vi "Read X.vi"(8 "error in (no error)":errorcluster, 11 "Vec3d Class in":refnum<class "Vec3d Class.lvclass">) -> (0 "error out":errorcluster, 2 "X":dbl, 3 "Vec3d Class out":refnum<class "Vec3d Class.lvclass">)   [LabVIEW 2011, in "Vec3d Class.lvclass"]
uses:
  Vec3d Class.lvclass
  Vec3d Class.lvclass/Vec3d Class.ctl
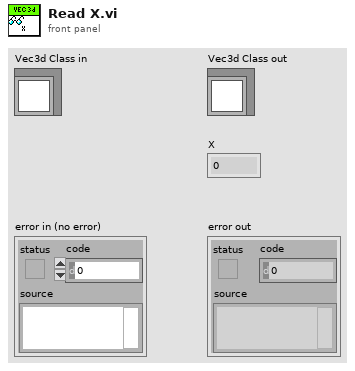
[diagram p1: front panel]
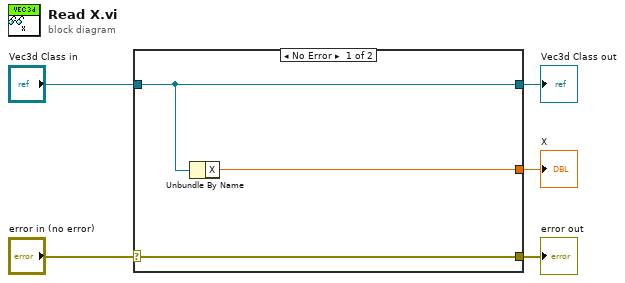
[diagram p0: block diagram]
diagram:
  n1 = case shown="No Error" "error in (no error)" {
    selector: "error in (no error)" -> [w8 w9]
    tunnel: [w8 w9] -> w4
    tunnel: [w7 w10] -> w2
    tunnel: "Vec3d Class in" -> [w7 w10]
    tunnel: [w6 _] -> w1
    frame No Error {
      n2 = Unbundle By Name(w7) -> ("X"=w6:dbl)
    }
    frame Error {
    }
  }
  "error out" <- w4
  "Vec3d Class out" <- w2
  "X" <- w1
